vi "Drawmatrix(SubVI).vi"(6 "Numeric":i32, 7 "Real Matrix (Column Vector)":T1, 9 "L - length":i32, 10 "D - width":i32, 11 "empty picture in":picture) -> (3 "empty picture out":picture)   [LabVIEW 2018]
uses:
  <vilib>/Analysis/Matrix/Datatypes/RealMatrix.ctl
  <vilib>/Analysis/Matrix/NI_Matrix.lvlib
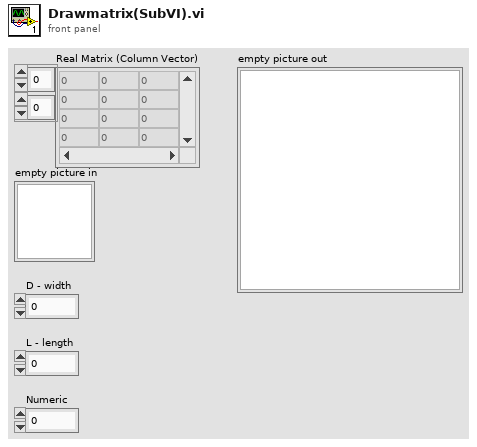
[diagram p1: front panel]
types:
  T1 = typedef "NI_Matrix.lvlib/RealMatrix.ctl" = dbl[][]
  T2 = cluster{"Width":u16, "Style":enum32{"Solid", "Dash", "Dot", "DashDot", "DashDotDot"}}
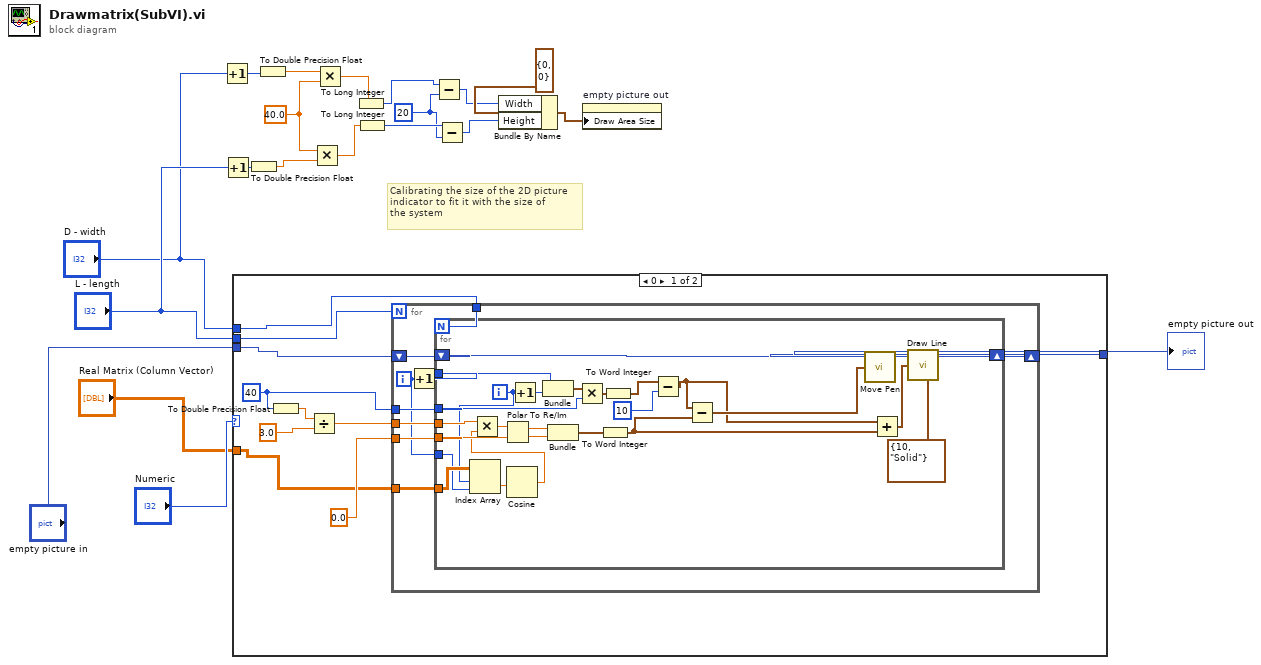
[diagram p0: block diagram]
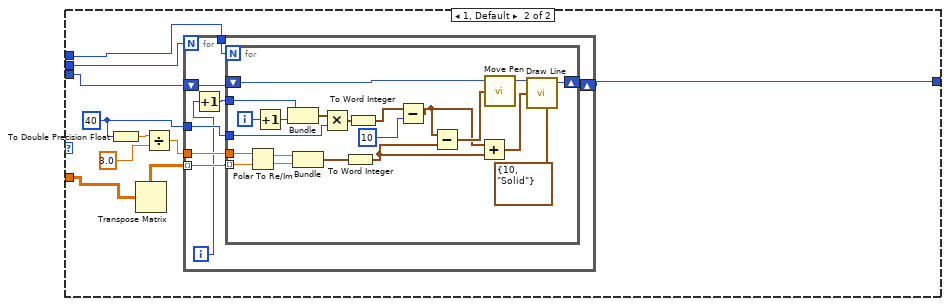
[diagram p2: hidden frame]
diagram:
  w5 = 20 ("y")
  w16 = 40.0 ("y")
  # "Calibrating the size of the 2D picture\nindicator to fit it with the size of\nthe system"
  n1 = Increment(x="D - width") -> (x+1=w13:i32)
  n2 = Increment(x="L - length") -> (x+1=w14:i32)
  n3 = case shown="0" "Numeric" {
    tunnel: [w27 w73] -> w17
    tunnel: "D - width" -> [w26 w71]
    tunnel: "L - length" -> [w25 w70]
    tunnel: "empty picture in" -> [w24 w72]
    tunnel: "Real Matrix (Column Vector)" -> [w21 w69]
    frame 0 {
      w28 = 40
      n4 = To Double Precision Float(number=w28) -> (double precision float=w29:dbl)
      n5 = Divide(x=w29, y=3.0) -> (x/y=w22:dbl)
      n6 = for {
        N: w25 -> [_]
        shift-right: [w38] -> w27
        shift-left: w24 -> [w39]
        tunnel: 0.0 -> [w36]
        tunnel: w26 -> [w35]
        tunnel: w28 -> [w34]
        tunnel: w22 -> [w33]
        tunnel: w21 -> [w32]
        i -> [w31]
        n7 = Increment(x=w31) -> (x+1=w37:i32)
        n8 = for {
          N: w35 -> [_]
          shift-right: [w57] -> w38
          shift-left: w39 -> [w61]
          tunnel: w37 -> [w56]
          tunnel: w36 -> [w52]
          tunnel: w34 -> [w51]
          tunnel: w33 -> [w46]
          tunnel: w32 -> [w44]
          tunnel: w31 -> [w43]
          i -> [w42]
          n9 = Index Array(array=w44, index (row)=w42, index (col)=w43) -> (element=w41:dbl)
          n10 = Cosine(x=w41) -> (cos(x)=w40:dbl)
          n11 = Multiply ("Multiply.vi")(x=w46, y=w40) -> (x*y=w45:dbl)
          n12 = Polar To Re/Im(2:w52, 3:w45) -> (0:w59:dbl, 1:w60:dbl)
          n13 = Increment(x=w42) -> (x+1=w55:i32)
          n14 = Bundle(w56, w55) -> (w63:cluster{i32, i32})  [unwired: 1 in]
          n15 = Bundle(w60, w59) -> (w58:cluster{dbl, dbl})  [unwired: 1 in]
          n16 = Multiply(x=w63, y=w51) -> (x*y=w54:cluster{i32, i32})
          n17 = To Word Integer(number=w58) -> (16bit integer=w53:cluster{i16, i16})
          n18 = To Word Integer(number=w54) -> (16bit integer=w49:cluster{i16, i16})
          n19 = Subtract(x=w49, y=10) -> (x-y=w47:cluster{i32, i32})
          n20 = Subtract(x=w47, y=w53) -> (x-y=w64:cluster{i32, i32})
          n21 = call <vilib>:"Move Pen.vi"("new position"=w64, "picture"=w61) -> ("new picture"=w65:picture)  [unwired: 3 in]
          n22 = Add(x=w47, y=w53) -> (x+y=w62:cluster{i32, i32})
          n23 = call <vilib>:"Draw Line.vi"("picture"=w65, "end point"=w62, "pen"=T2 {"Width"=10, "Style"=enum."Solid"}) -> ("new picture"=w57:picture)  [unwired: 6 in]
        }
      }
    }
    frame 1, Default {
      w67 = 40
      n24 = To Double Precision Float(number=w67) -> (double precision float=w74:dbl)
      n25 = Transpose Matrix(1:w69) -> (0:w68:T1)
      n26 = Divide(x=w74, y=3.0) -> (x/y=w66:dbl)
      n27 = for {
        N: w70 -> [_]
        shift-right: [w82] -> w73
        shift-left: w72 -> [w81]
        tunnel: w71 -> [w80]
        tunnel: w68 -> [w79] mode=indexing
        tunnel: w67 -> [w78]
        tunnel: w66 -> [w77]
        i -> [w76]
        n28 = Increment(x=w76) -> (x+1=w83:i32)
        n29 = for {
          N: w80 -> [_]
          shift-right: [w96] -> w82
          shift-left: w81 -> [w100]
          tunnel: w83 -> [w95]
          tunnel: w79 -> [w90] mode=indexing
          tunnel: w78 -> [w89]
          tunnel: w77 -> [w88]
          i -> [w94]
          n30 = Polar To Re/Im(2:w90, 3:w88) -> (0:w98:dbl, 1:w99:dbl)
          n31 = Increment(x=w94) -> (x+1=w93:i32)
          n32 = Bundle(w95, w93) -> (w102:cluster{i32, i32})  [unwired: 1 in]
          n33 = Bundle(w99, w98) -> (w97:cluster{dbl, dbl})  [unwired: 1 in]
          n34 = Multiply(x=w102, y=w89) -> (x*y=w92:cluster{i32, i32})
          n35 = To Word Integer(number=w97) -> (16bit integer=w91:cluster{i16, i16})
          n36 = To Word Integer(number=w92) -> (16bit integer=w86:cluster{i16, i16})
          n37 = Subtract(x=w86, y=10) -> (x-y=w84:cluster{i32, i32})
          n38 = Subtract(x=w84, y=w91) -> (x-y=w103:cluster{i32, i32})
          n39 = Add(x=w84, y=w91) -> (x+y=w101:cluster{i32, i32})
          n40 = call <vilib>:"Move Pen.vi"("new position"=w103, "picture"=w100) -> ("new picture"=w104:picture)  [unwired: 3 in]
          n41 = call <vilib>:"Draw Line.vi"("picture"=w104, "end point"=w101, "pen"=T2 {"Width"=10, "Style"=enum."Solid"}) -> ("new picture"=w96:picture)  [unwired: 6 in]
        }
      }
    }
  }
  "empty picture out" <- w17
  n42 = To Double Precision Float(number=w14) -> (double precision float=w15:dbl)
  n43 = To Double Precision Float(number=w13) -> (double precision float=w12:dbl)
  n44 = Multiply(x=w16, y=w15) -> (x*y=w4:dbl)
  n45 = Multiply(x=w12, y=w16) -> (x*y=w3:dbl)
  n46 = To Long Integer(number=w3) -> (32bit integer=w8:i32)
  n47 = To Long Integer(number=w4) -> (32bit integer=w6:i32)
  n48 = Subtract(x=w8, y=w5) -> (x-y=w7:i32)
  n49 = Subtract(x=w6, y=w5) -> (x-y=w9:i32)
  n50 = Bundle By Name(cluster=cluster{"Height":u32, "Width":u32} {"Height"=0, "Width"=0} ("input cluster"), "Width"=w7, "Height"=w9) -> (w11:cluster{"Height":u32, "Width":u32})
  n51 = property on="empty picture out" class="Pict"("Draw Area Size"=w11) -> ()  [unwired: 2 in, 2 out]
